vi "Wait For DAQ to Stop.vi"(8 "error in (no error)":errorcluster, 10 "timeout (ms)":i32=5000) -> (0 "error out":errorcluster={"status"=FALSE, "code"=0, "source"="."})   [LabVIEW 2020]
doc: "Waits for the DAQ thread to terminate execution. If another measurement is to be started immediately, it is important to wait for the first to finish to avoid conflicts."
uses:
  PXI Globals.vi
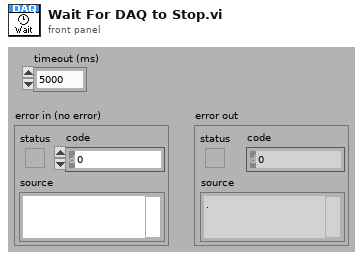
[diagram p1: front panel]
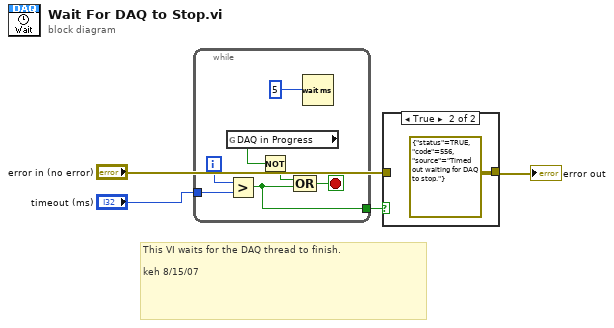
[diagram p0: block diagram]
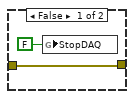
[diagram p2: hidden frame]
diagram:
  # "This VI waits for the DAQ thread to finish.\n\nkeh 8/15/07"
  n1 = while {
    tunnel: "timeout (ms)" -> [w6]
    tunnel: [w7] -> w1
    i -> [w8]
    stop <- w10 stop-if-true
    n2 = global read "PXI Globals.vi" "DAQ in Progress"() -> (w9:bool)
    n3 = Greater?(x=w8, y=w6) -> (0:w7:bool)
    n4 = Not(x=w9) -> (.not. x?=w5:bool)
    n5 = Compound Arithmetic op=OR(w5, w7) -> (w10:bool)
    n6 = Wait (ms)(milliseconds to wait=5) -> ()  [unwired: 1 out]
  }
  n7 = case shown="True" w1 {
    tunnel: [w13 errorcluster {"status"=TRUE, "code"=556, "source"="Timed out waiting for DAQ to stop."} ("error out 2")] -> w4
    tunnel: "error in (no error)" -> [w13 _]
    frame False {
      n8 = global write "PXI Globals.vi" "StopDAQ"(FALSE ("StopDAQ")) -> ()
    }
    frame True {
    }
  }
  "error out" <- w4
